vi "PLC傳值讀值超過65535_2.vi"(0 "Read PLC Reg Index0":i32=50, 1 "Input Registers":u16[](array[numeric])=[0, 0, 0, 0, 0, 0, 0, 0], 5 "Read PLC Reg Index1":i32=50, 7 "Out輸入值":u32=130000, 9 "Out starting address":u16=260, 11 "error in (no error)":errorcluster, 12 "Enum":enum16{"Send PLC Data", "Receive PLC Data"}(ring)) -> (4 "Receive PLC Data":i32, 6 "Receive PLC Data":string, 15 "error out":errorcluster)   [LabVIEW 2019]
uses:
  Ctrl/ModbusCmd.ctl
panel:
  out "(hi.lo)":u32
  out "output array":i32[](array[numeric])
  out "lo(x)":u16
  out "hi(x)":u16
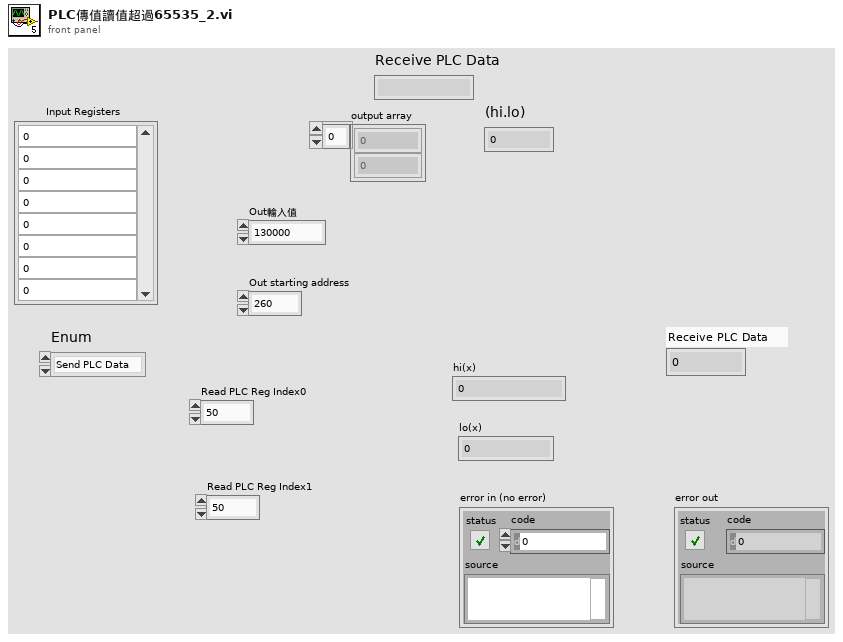
[diagram p1: front panel]
types:
  T1 = cluster{"starting address":u16, "number of inputs":u16, "Sat Coils":bool[], "Holding Registers":u16[]}
  T2 = typedef "ModbusCmd.ctl" = enum16{"Connect", "Disconnect", "Init", "Fetch Basic Objects", "Fetch Input Refisters", "Fetch Discrete Inputs", "Set Coils", "Set Holding Registers", "Write Single Holding", "Exit"}
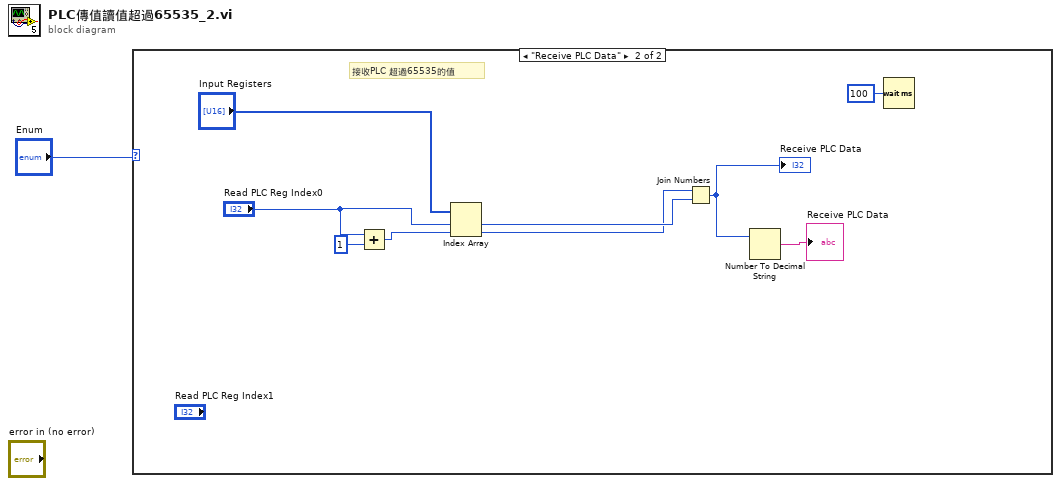
[diagram p0: block diagram]
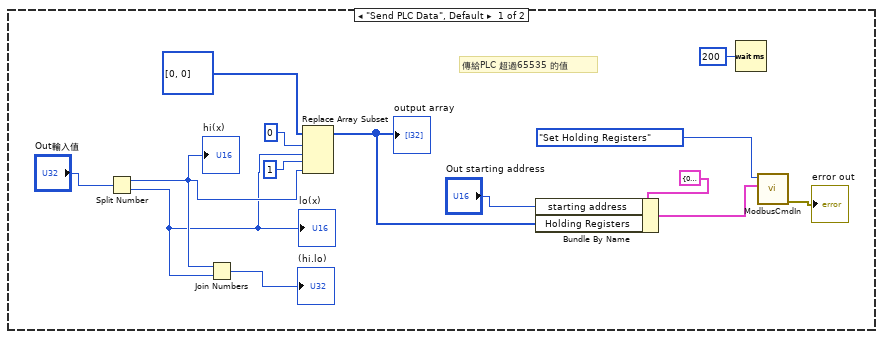
[diagram p2: hidden frame]
diagram:
  n1 = case shown="\"Receive PLC Data\"" "Enum" {
    frame "Send PLC Data", Default {
      # "傳給PLC 超過65535 的值"
      n2 = Split Number(x="Out輸入值") -> (hi(x)=w5:u16, lo(x)=w4:u16)
      "hi(x)" <- w5
      "lo(x)" <- w4
      n3 = Join Numbers(hi=w5, lo=w4) -> ((hi.lo)=→"(hi.lo)":u32)
      n4 = Replace Array Subset(array=i32[] [0, 0], new element #1=w4, index #1=0 ("index"), new element #2=w5, index #2=1 ("index")) -> (w13:i32[])
      "output array" <- w13
      n5 = Bundle By Name(cluster=T1 {"starting address"=0, "number of inputs"=0, "Sat Coils"=[FALSE], "Holding Registers"=[]} ("data"), "starting address"="Out starting address", "Holding Registers"=w13) -> (w11:T1)
      n6 = Wait (ms)(milliseconds to wait=u32 200) -> ()  [unwired: 1 out]
      n7 = call "ModbusCmdIn.vi"("data"=w11, "Enum"=ModbusCmd."Set Holding Registers") -> ("error out"=→"error out":errorcluster)  [unwired: 9 in]
    }
    frame "Receive PLC Data" {
      # "接收PLC 超過65535的值"
      n8 = Add(x="Read PLC Reg Index0", y=1) -> (x+y=w18:i32)
      n9 = Index Array(array="Input Registers", index #1="Read PLC Reg Index0", index #2=w18) -> (element #1=w24:u16, element #2=w16:u16)
      n10 = Join Numbers(hi=w16, lo=w24) -> ((hi.lo)=w23:u32)
      "Receive PLC Data" <- w23
      n11 = Number To Decimal String(number=w23) -> (decimal integer string=→"Receive PLC Data":string)  [unwired: 1 in]
      n12 = Wait (ms)(milliseconds to wait=u32 100) -> ()  [unwired: 1 out]
    }
  }
